vi "flat.vi"(11 "Input":dbl[](array[numeric])) -> (3 "XY Graph 3":cluster{dbl[], dbl[]}(graph))   [LabVIEW 2014]
uses:
  <vilib>/Analysis/6fits.llb/Curve Fitting Criteria.ctl
  <vilib>/Analysis/baseanly.llb/Real A x B.vi
  <vilib>/Analysis/NI_AALPro.lvlib
  <vilib>/Analysis/NI_AALBase.lvlib
panel:
  out "XY Graph 2":cluster{dbl[], dbl[]}(graph)
  out "slope":dbl caption="기울기"
  out "XY Graph":cluster{dbl[], dbl[]}(graph)
  in  "time":dbl[](array[numeric])=[1.0, 2.0, 3.0, 4.0, 5.0, 6.0, 7.0, 8.0, 9.0, 10.0, 11.0, 12.0, 13.0, 14.0, 15.0, 16.0, 17.0, 18.0, 19.0, 20.0, 21.0, 22.0, 23.0, 24.0]
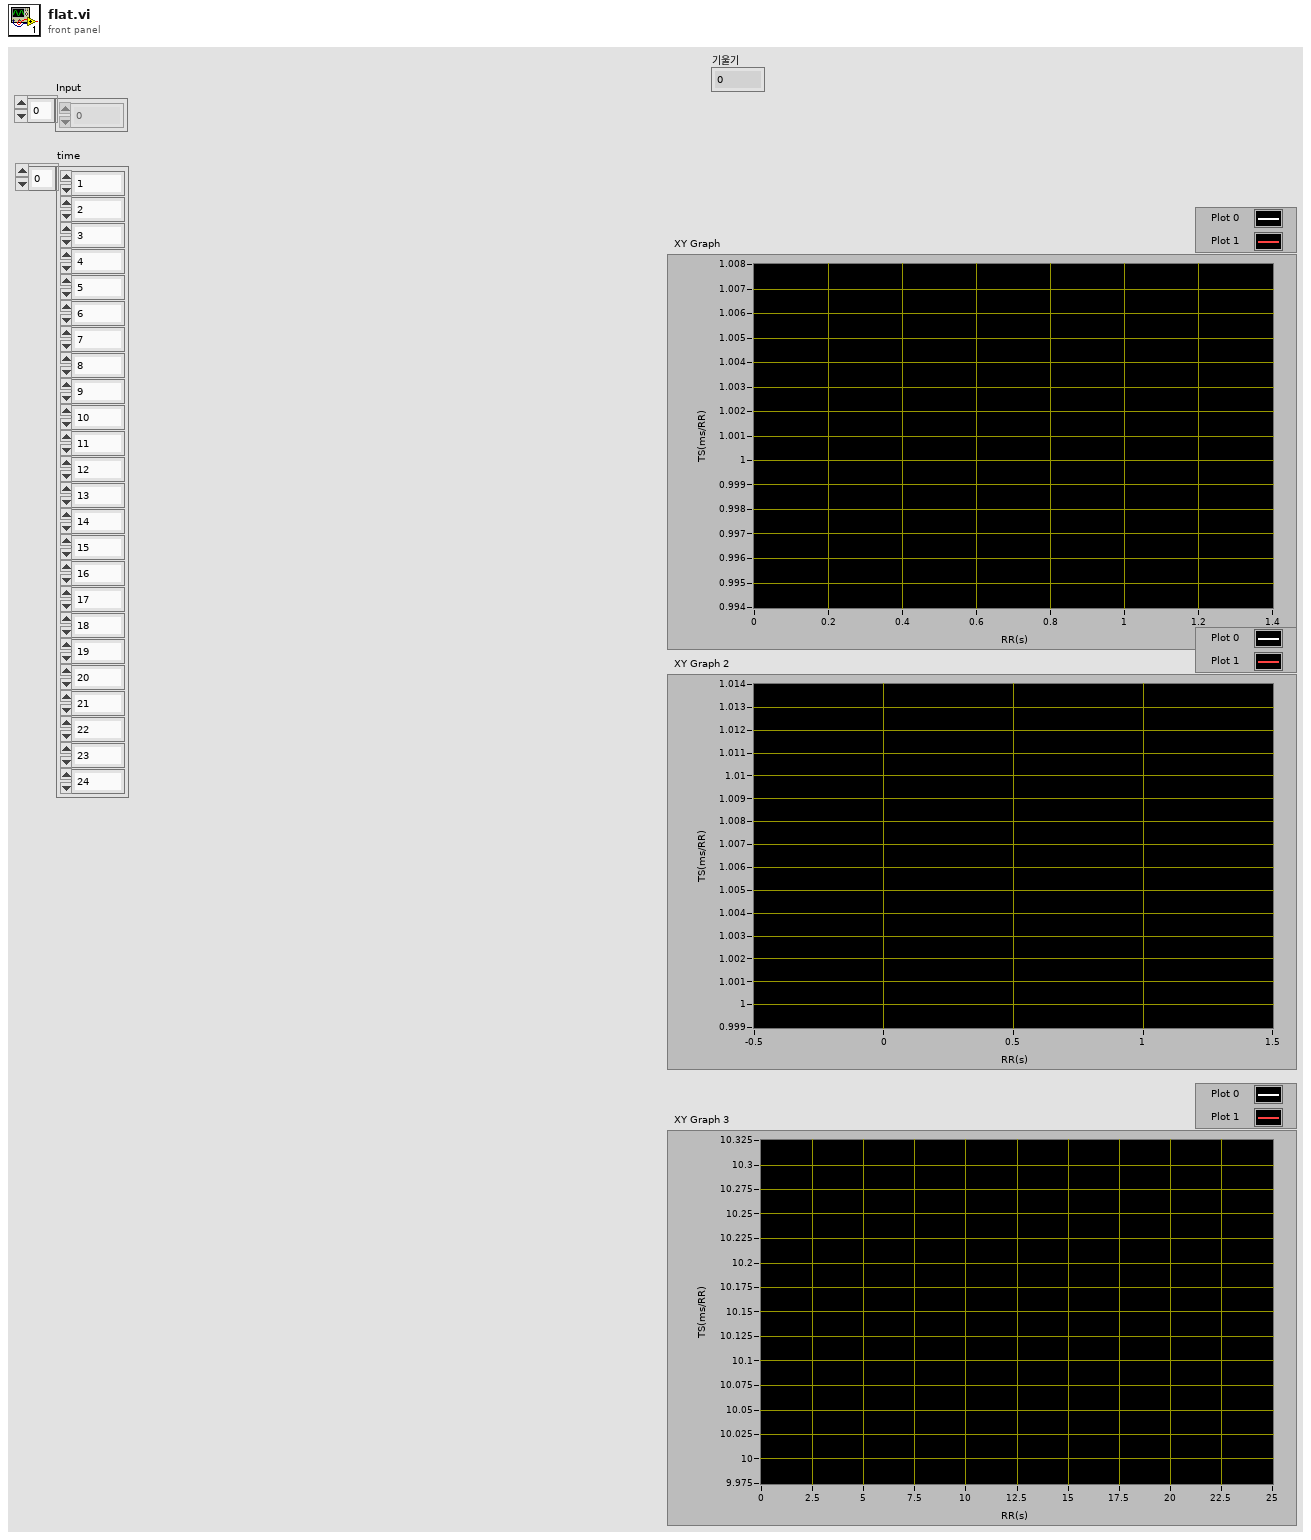
[diagram p1: front panel]
types:
  T1 = typedef "NI_AALPro.lvlib/Curve Fitting Criteria.ctl" = u16
  T2 = typedef "NI_Matrix.lvlib/RealMatrix.ctl" = dbl[][]
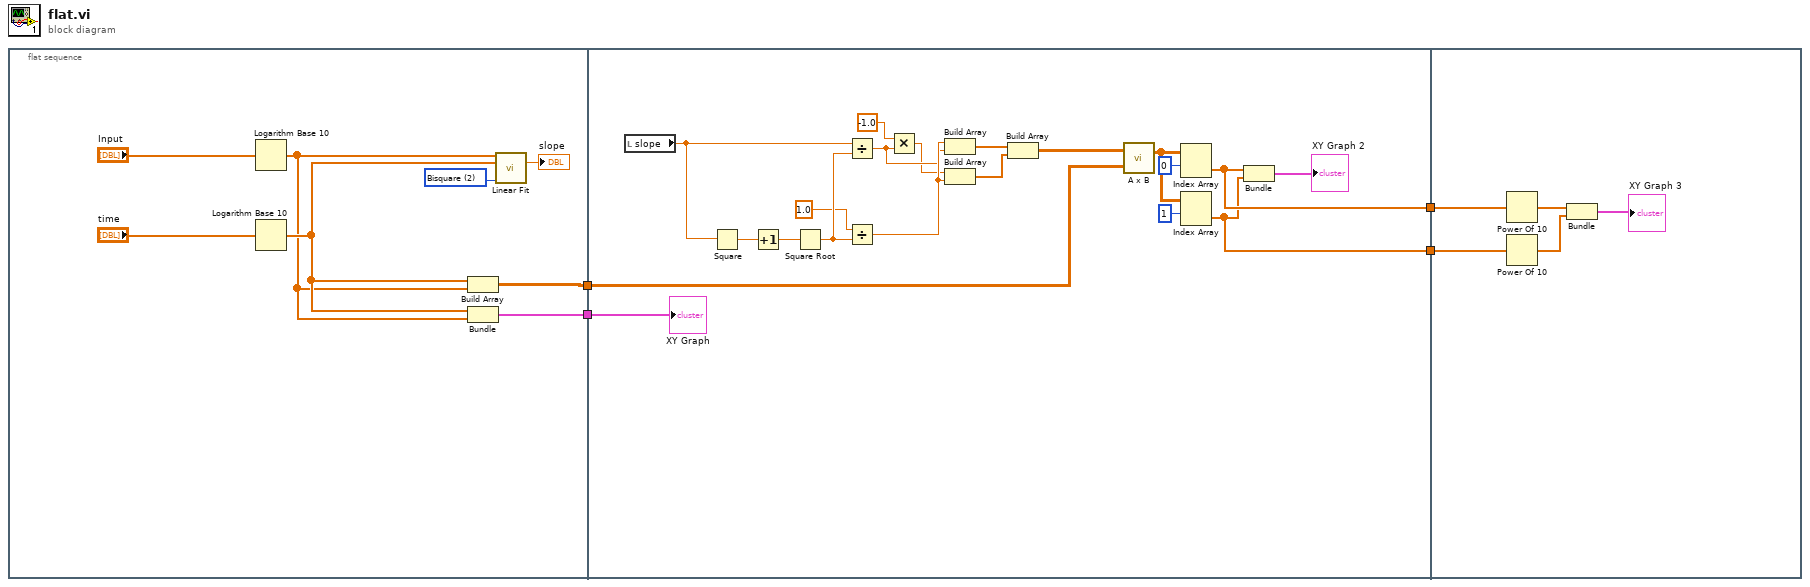
[diagram p0: block diagram]
diagram:
  n1 = flat-sequence {
    tunnel: [w9] -> w4
    tunnel: [w5] -> w3
    tunnel: w4 -> [w32]
    tunnel: w3 -> [w21]
    tunnel: [w14] -> w2
    tunnel: [w13] -> w1
    tunnel: w2 -> [w37]
    tunnel: w1 -> [w36]
    frame #0 {
      w11 = T1 2 items=["Least Square", "Least Absolute Residual", "Bisquare"] ("method")
      n2 = Logarithm Base 10(1:"Input") -> (0:w6:dbl[])
      n3 = Logarithm Base 10(1:"time") -> (0:w7:dbl[])
      n4 = Build Array(w7, w6) -> (w5:dbl[][])
      n5 = Bundle(w7, w6) -> (w9:cluster{dbl[], dbl[]})  [unwired: 1 in]
      n6 = call <vilib>:"Linear Fit.vi"("Y"=w6, "X"=w7, "method"=w11) -> ("slope"=→"slope":dbl)  [unwired: 8 in, 4 out]
    }
    frame #1 {
      n7 = local read "slope"() -> (w28:dbl)
      n8 = Square(x=w28) -> (x^2=w31:dbl)
      n9 = Increment(x=w31) -> (x+1=w30:dbl)
      n10 = Square Root(x=w30) -> (sqrt(x)=w29:dbl)
      n11 = Divide(x=w28, y=w29) -> (x/y=w16:dbl)
      n12 = Divide(x=1.0, y=w29) -> (x/y=w25:dbl)
      n13 = Multiply(x=-1.0, y=w16) -> (x*y=w15:dbl)
      n14 = Build Array(w25, w16) -> (w24:dbl[])
      n15 = Build Array(w15, w25) -> (w23:dbl[])
      n16 = Build Array(w24, w23) -> (w22:dbl[][])
      n17 = call-poly <vilib>:"A x B.vi"("B"=w21, "A"=w22) -> ("A x B"=w20:T2)  [unwired: 1 out]
      n18 = Index Array(array=w20, index (row)=0 ("인덱스 (행)")) -> (element=w14:dbl[])  [unwired: 1 in]
      n19 = Index Array(array=w20, index (row)=1 ("인덱스 (행)")) -> (element=w13:dbl[])  [unwired: 1 in]
      n20 = Bundle("A x B"=w14, "A x B"=w13) -> (→"XY Graph 2":cluster{"A x B":dbl[], "A x B":dbl[]})  [unwired: 1 in]
      "XY Graph" <- w32
    }
    frame #2 {
      n21 = Power Of 10(x=w37) -> (10^x=w35:dbl[])
      n22 = Power Of 10(x=w36) -> (10^x=w34:dbl[])
      n23 = Bundle(w35, w34) -> (→"XY Graph 3":cluster{dbl[], dbl[]})  [unwired: 1 in]
    }
  }
